vi "registerSubscriber_old.vi"(1 "Parameters":T2={"Caller ID"="/ChrisAir", "Topic"="/robot/joint_states", "Topic Type"="sensor_msgs/JointState", "Caller API"="http://192.168.1.111"}) -> (2 "Error out":errorcluster, 3 "Reply":T1={"Code"=1, "statusMessage"="Subscribed to [/robot/joint_states]", "APIs"=["http://tuftsBaxter.local:60639/"]}, 4 "Reply":string="HTTP/1.0 200 OK\r\nServer: BaseHTTP/0.3 Python/2.7.1\r\nDate: Fri, 31 May 2013 11:54:05 GMT\r\nContent-type: text/xml\r\nContent-length: 343\r\n\r\n<?xml version='1.0'?>\n<methodResponse>\n<params>\n<param>\n<value><array><data>\n<value><int>1</int></value>\n<value><string>Subscribed to [/robot/joint_states]</string></value>\n<value><array><data>\n<value><string>http://tuftsBaxter.local:60639/</string></value>\n</data></array></value>\n</data></array></value>\n</param>\n</params>\n</methodResponse>\n", 5 "registerSubscriber":string="POST /RPC2 HTTP/1.1\r\nHost: 192.168.1.110:11311\r\nContent-Type: text/xml\r\nContent-Length: 396\r\n\r\n<?xml version='1.0'?>\n<methodCall>\r <methodName>registerSubscriber</methodName>\r <params>\r   <param><value><string>/ChrisAir</string> </value> </param>\r   <param><value><string>/robot/joint_states</string> </value> </param>\r   <param><value><string>sensor_msgs/JointState</string> </value> </param>\r   <param><value><string>http://192.168.1.111</string> </value> </param>\r </params>\r</methodCall>")   [LabVIEW 2013]
uses:
  _ROSDefinition.vi
panel:
  out "Replies":string[](array[string])=["HTTP/1.1 200 OK\r\nServer: XMLRPC++ 0.7\r\nContent-Type: text/xml\r\nContent-length: 303\r\n\r\n<?xml version=\"1.0\"?>\r\n<methodResponse><params><param>\r\n\t<value><array><data><value><i4>1</i4></value><value></value><value><array><data><value>TCPROS</value><value>tuftsBaxter.local</value><value><i4>58491</i4></value></data></array></value></data></array></value>\r\n</param></params></methodResponse>\r\n"]
  out "ports":string[](array[string])=["http://tuftsBaxter.local:60639/"]
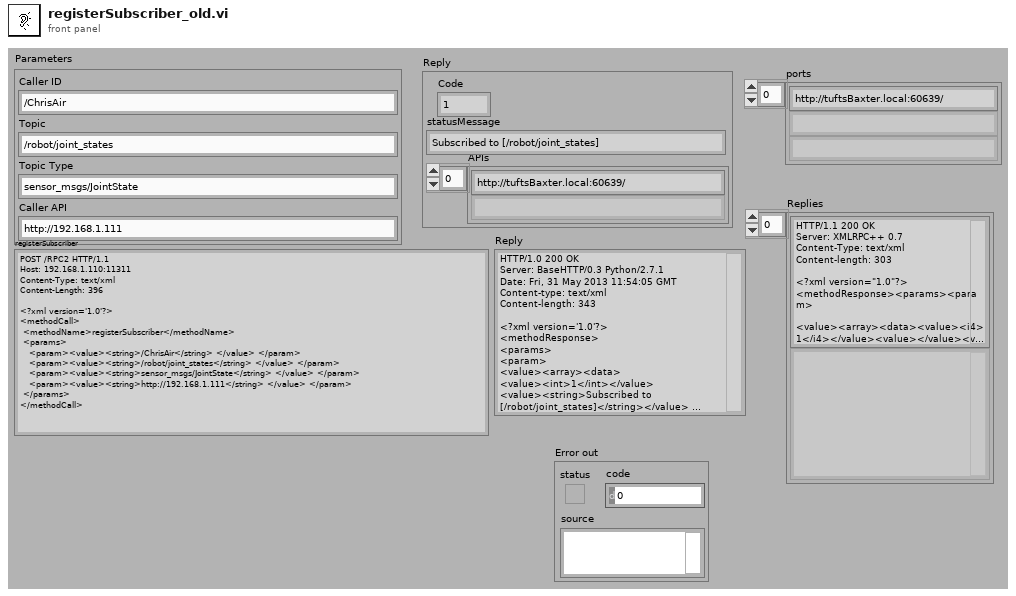
[diagram p1: front panel]
types:
  T1 = cluster{"Code":i8, "statusMessage":string, "APIs":string[]}
  T2 = cluster{"Caller ID":string, "Topic":string, "Topic Type":string, "Caller API":string}
  T3 = cluster{"Code":i8, "statusMessage":string, "APIs":string[]}[]
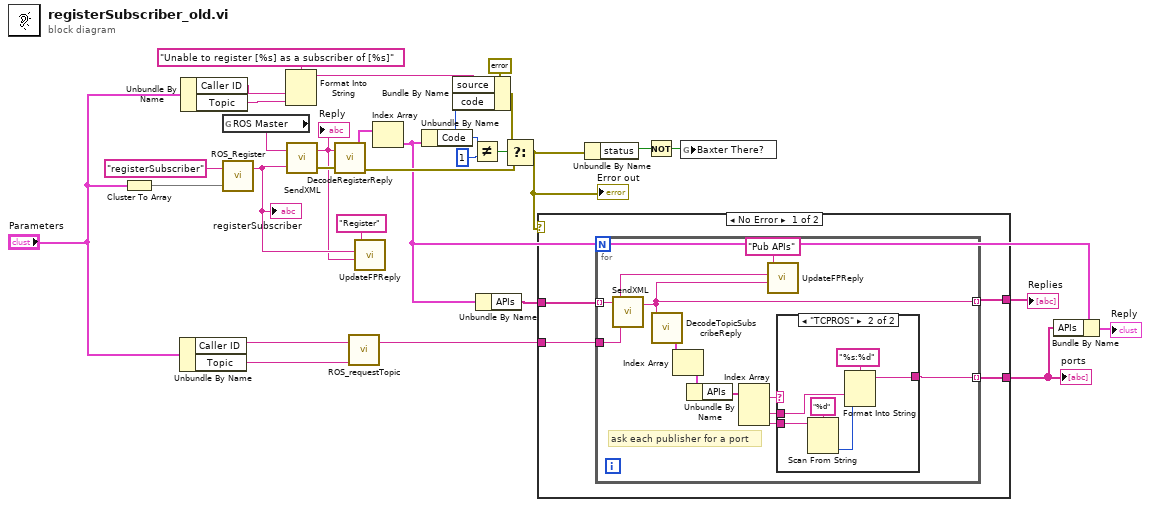
[diagram p0: block diagram]
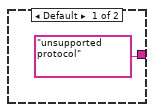
[diagram p2: hidden frame]
diagram:
  n1 = Cluster To Array(cluster="Parameters") -> (array=w4:string[])
  n2 = Unbundle By Name("Parameters") -> ("Caller ID"=w13:string, "Topic"=w12:string)
  n3 = Unbundle By Name("Parameters") -> ("Caller ID"=w27:string, "Topic"=w28:string)
  n4 = global read "_ROSDefinition.vi" "ROS Master"() -> (w29:string)
  n5 = call "ROS_Register.vi"("Parameters"=w4, "Method Name"="registerSubscriber") -> ("registerSubscriber"=w2:string)  [unwired: 1 in]
  "registerSubscriber" <- w2
  n6 = Format Into String(format string="Unable to register [%s] as a subscriber of [%s]" ("source"), w27, w28) -> (resulting string=w17:string)  [unwired: 2 in, 1 out]
  n7 = call "SendXML.vi"("Send"=w2, "URI in"=w29) -> ("error out"=w23:errorcluster, "Reply"=w1:string)
  "Reply" <- w1
  n8 = call "DecodeRegisterReply.vi"("error in (no error)"=w23, "Response"=w1) -> ("error out"=w19:errorcluster, "Reply"=w22:T3)
  n9 = call "ROS_requestTopic.vi"("Topic"=w12, "Caller ID"=w13) -> ("XML"=w11:string)  [unwired: 1 in]
  n10 = call "UpdateFPReply.vi"("Reply"=w1, "Sent"=w2, "method"="Register" ("name (unnamed)")) -> ()  [unwired: 3 in]
  n11 = Index Array(array=w22) -> (element=w9:T1)  [unwired: 1 in]
  n12 = Unbundle By Name(w9) -> ("Code"=w16:i8)
  n13 = Bundle By Name(cluster=errorcluster {"status"=TRUE, "code"=0, "source"=" Error"} ("t"), "source"=w17, "code"=w16) -> (w15:errorcluster)
  n14 = Not Equal?(x=w16, y=i8 1) -> (x != y?=w20:bool)
  n15 = Unbundle By Name(w9) -> ("APIs"=w14:string[])
  n16 = Select(t=w15, s=w20, f=w19) -> (s? t:f=w6:errorcluster)
  "Error out" <- w6
  n17 = case shown="No Error" w6 {
    tunnel: w14 -> [w34 _]
    tunnel: w11 -> [w33 _]
    tunnel: [w32 _] -> w10
    tunnel: [w31 _] -> w8
    frame No Error {
      n18 = for {
        tunnel: w34 -> [w37] mode=indexing
        tunnel: [w35] -> w32 mode=indexing
        tunnel: w33 -> [w36]
        tunnel: [w45] -> w31 mode=indexing
        # "ask each publisher for a port"
        n19 = call "SendXML.vi"("Send"=w36, "URI in"=w37) -> ("Reply"=w35:string)  [unwired: 1 out]
        n20 = call "DecodeTopicSubscribeReply.vi"("Topic Reply"=w35) -> ("Reply"=w44:T3)  [unwired: 1 in, 1 out]
        n21 = Index Array(array=w44) -> (element=w43:T1)  [unwired: 1 in]
        n22 = Unbundle By Name(w43) -> ("APIs"=w42:string[])
        n23 = Index Array(array=w42) -> (element #1=w39:string, element #2=w41:string, element #3=w40:string)  [unwired: 3 in]
        n24 = call "UpdateFPReply.vi"("Reply"=w35, "Sent"=w36, "method"="Pub APIs" ("name (unnamed)")) -> ()  [unwired: 3 in]
        n25 = case shown="\"TCPROS\"" w39 {
          tunnel: ["unsupported protocol" w51] -> w45
          tunnel: w41 -> [_ w50]
          tunnel: w40 -> [_ w49]
          frame Default {
          }
          frame "TCPROS" {
            n26 = Scan From String(format string="%d", input string=w49) -> (output 1=w48:i32)  [unwired: 3 in, 3 out]
            n27 = Format Into String(format string="%s:%d", w50, w48) -> (resulting string=w51:string)  [unwired: 2 in, 1 out]
          }
        }
      }
    }
    frame Error {
    }
  }
  "ports" <- w8
  "Replies" <- w10
  n28 = Unbundle By Name(w6) -> ("status"=w24:bool)
  n29 = Not(x=w24) -> (.not. x?=w25:bool)
  n30 = global write "_ROSDefinition.vi" "Baxter There?"(w25) -> ()
  n31 = Bundle By Name(cluster=w9, "APIs"=w8) -> (→"Reply":T1)
